vi "Chirp_fit.vi"() -> ()   [LabVIEW 2009]
panel:
  in  "Chirp up to (GHz)":dbl
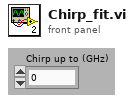
[diagram p1: front panel]
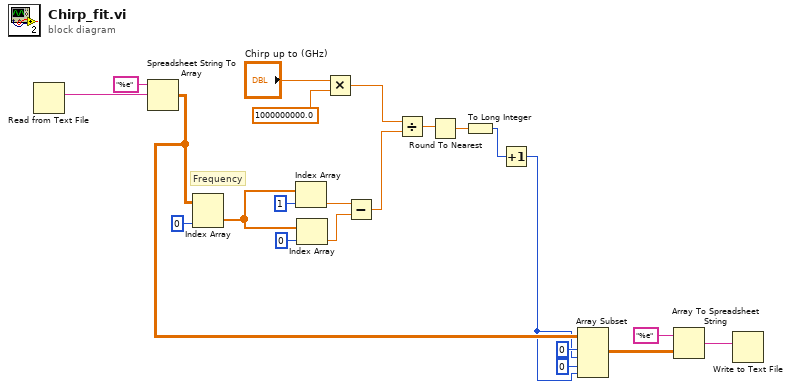
[diagram p0: block diagram]
diagram:
  # "Frequency"
  n1 = Read from Text File() -> (text=w22:string)  [unwired: 4 in, 3 out]
  n2 = Spreadsheet String To Array(format string="%e", spreadsheet string=w22) -> (array=w6:dbl[][])  [unwired: 2 in]
  n3 = Index Array(array=w6, index (col)=0 ("disabled index (col)")) -> (element=w17:dbl[])  [unwired: 1 in]
  n4 = Index Array(array=w17, index=1) -> (element=w14:dbl)
  n5 = Index Array(array=w17, index=0) -> (element=w13:dbl)
  n6 = Multiply(x="Chirp up to (GHz)", y=1000000000.0) -> (x*y=w10:dbl)
  n7 = Subtract(x=w14, y=w13) -> (x-y=w9:dbl)
  n8 = Divide(x=w10, y=w9) -> (x/y=w8:dbl)
  n9 = Round To Nearest(number=w8) -> (nearest integer value=w7:dbl)
  n10 = To Long Integer(number=w7) -> (32bit integer=w3:i32)
  n11 = Increment(x=w3) -> (x+1=w2:i32)
  n12 = Array Subset(array=w6, index (row)=0 ("index"), length (row)=w2, index (col)=0 ("index"), length (col)=w2) -> (w1:dbl[][])
  n13 = Array To Spreadsheet String(array=w1, 3:"%e" ("format string")) -> (spreadsheet string=w20:string)  [unwired: 1 in]
  n14 = Write to Text File(text=w20) -> ()  [unwired: 3 in, 3 out]
